vi "Process Command.vi"(8 "error in":errorcluster, 10 "message in":T1, 11 "lia rt in":refnum<class "Lock-In Amplifier Example RT.lvclass">) -> (0 "error out":errorcluster, 1 "send response":bool, 2 "message out":T1, 3 "lia rt out":refnum<class "Lock-In Amplifier Example RT.lvclass">)   [LabVIEW 2017, in "Lock-In Amplifier Example RT.lvclass"]
uses:
  Lock-In Amplifier Example RT.lvclass
  shared/Public/message.ctl
  host/Public/lock-in settings.ctl
  host/Public/pll settings.ctl
  Properties/FpgaSession_GET.vi
  interface/Interface FPGA/Properties/FpgaSession_GET.vi
  interface/Interface FPGA/LIA Host Interface FPGA.lvclass
  host/Lock-In Amplifier Example Host.lvlib
  shared/Lock-In Amplifier Example Shared.lvlib
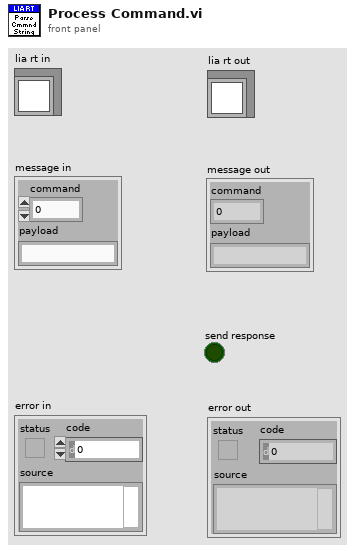
[diagram p1: front panel]
types:
  T1 = typedef "Lock-In Amplifier Example Shared.lvlib/message.ctl" = cluster{"command":u32, "payload":string}
  T2 = typedef "Lock-In Amplifier Example Host.lvlib/lock-in settings.ctl" = cluster{"decimation":i32, "source":i32, "carrier source":i32, "carrier":dbl}
  T3 = cluster{"instance":i32, "config":cluster{"config":T2, "record length":u32}}
  T4 = typedef "Lock-In Amplifier Example Host.lvlib/pll settings.ctl" = cluster{"source":i32, "q frequency":dbl}
  T5 = cluster{"instance":i32, "config":cluster{"carrier":dbl, "level":dbl}}
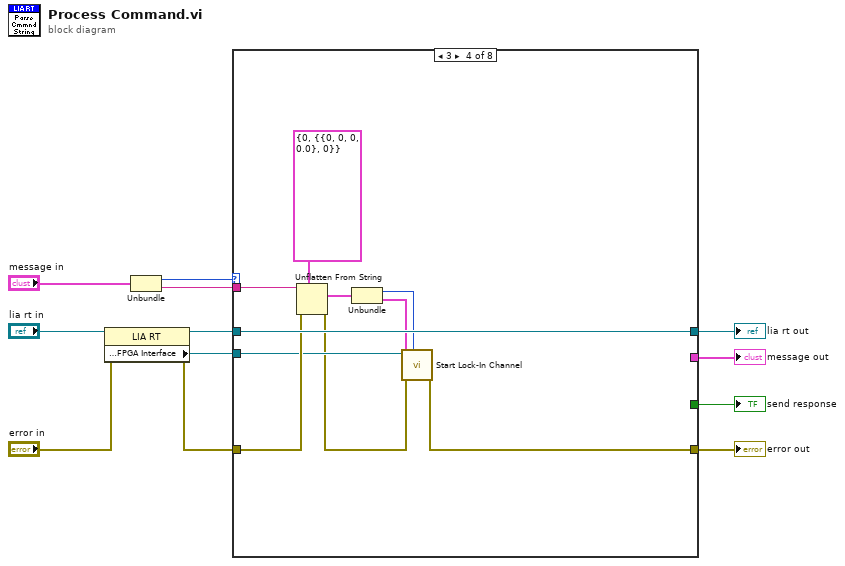
[diagram p0: block diagram]
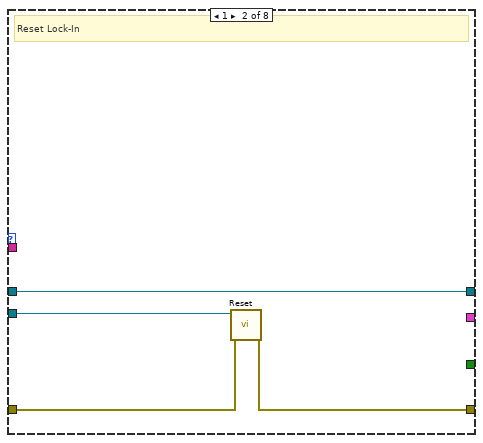
[diagram p3: hidden frame]
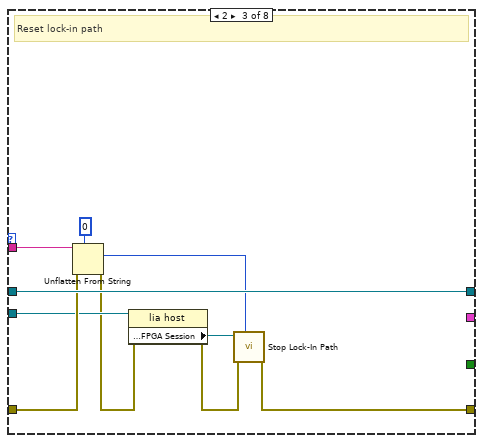
[diagram p4: hidden frame]
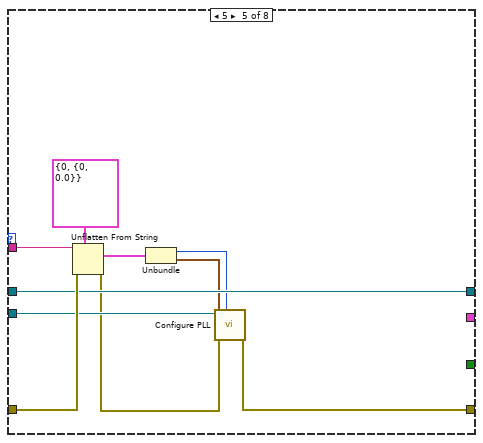
[diagram p5: hidden frame]
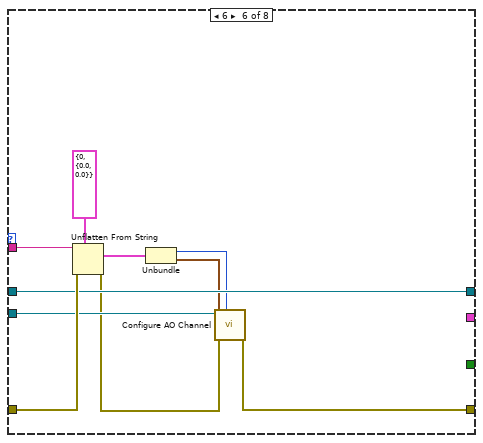
[diagram p6: hidden frame]
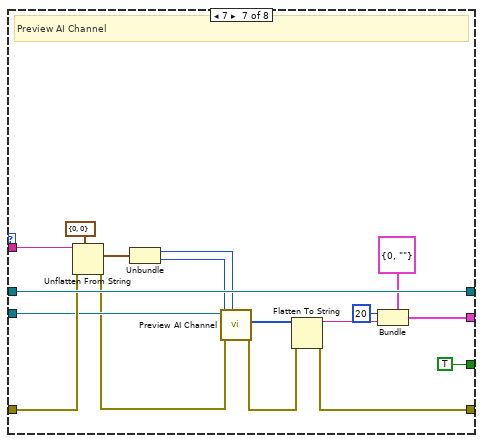
[diagram p7: hidden frame]
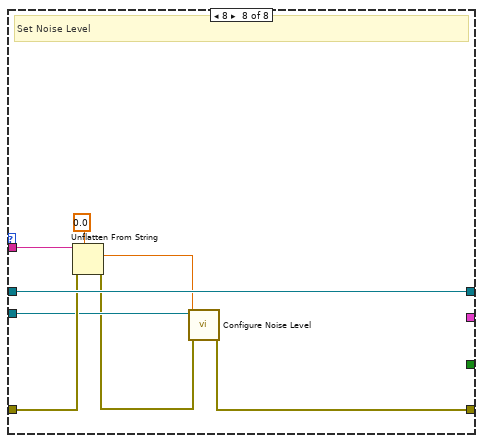
[diagram p8: hidden frame]
diagram:
  n1 = property class="LIA RT"(reference="lia rt in", error in="error in") -> (reference out=w8:refnum<class "Lock-In Amplifier Example RT.lvclass">, error out=w6:errorcluster, "Properties:FPGA Interface"=w5:refnum<class "LIA Host Interface FPGA.lvclass">)
  n2 = Unbundle("message in") -> ("command"=w11:u32, "payload"=w10:string)
  n3 = case shown="3" w11 {
    tunnel: w10 -> [_ _ w26 w37 w48 w58 w74 w82]
    tunnel: w8 -> [w14 w18 w28 w38 w43 w54 w75 w83]
    tunnel: w6 -> [w13 w16 w25 w36 w47 w57 w73 w81]
    tunnel: w5 -> [_ w17 w22 w35 w44 w55 w66 w80]
    tunnel: [w14 w18 w28 w38 w43 w54 w75 w83] -> w4
    tunnel: [w13 w15 w27 w33 w39 w51 w60 w76] -> w3
    tunnel: [_ _ _ _ _ _ w69 _] -> w2
    tunnel: [_ _ _ _ _ _ TRUE _] -> w1
    frame 0, Default {
    }
    frame 1 {
      # "Reset Lock-In"
      n4 = call-dynamic "Reset.vi"("error in"=w16, "host in"=w17) -> ("error out"=w15:errorcluster)  [unwired: 8 in, 1 out]
    }
    frame 2 {
      # "Reset lock-in path"
      n5 = Unflatten From String(type=0, binary string=w26, error in (no error)=w25) -> (value=w23:i32, error out=w21:errorcluster)  [unwired: 2 in, 1 out]
      n6 = property class="lia host"(reference=w22, error in=w21) -> (error out=w20:errorcluster, "Properties:FPGA Session"=w19:refnum<k20>)  [unwired: 1 out]
      n7 = call "Stop Lock-In Path.vi"("instance"=w23, "error in"=w20, "fpga session in"=w19) -> ("error out"=w27:errorcluster)  [unwired: 7 in, 1 out]
    }
    frame 3 {
      n8 = Unflatten From String(type=T3 {"instance"=0, "config"={"config"={"decimation"=0, "source"=0, "carrier source"=0, "carrier"=0.0}, "record length"=0}} ("output cluster"), binary string=w37, error in (no error)=w36) -> (value=w32:T3, error out=w34:errorcluster)  [unwired: 2 in, 1 out]
      n9 = Unbundle(w32) -> ("instance"=w31:i32, "config"=w30:cluster{"config":T2, "record length":u32})
      n10 = call-dynamic "Start Lock-In Channel.vi"("index"=w31, "error in"=w34, "config"=w30, "host in"=w35) -> ("error out"=w33:errorcluster)  [unwired: 6 in, 1 out]
    }
    frame 5 {
      n11 = Unflatten From String(type=cluster{"instance":i32, "config":T4} {"instance"=0, "config"={"source"=0, "q frequency"=0.0}}, binary string=w48, error in (no error)=w47) -> (value=w45:cluster{"instance":i32, "config":T4}, error out=w40:errorcluster)  [unwired: 2 in, 1 out]
      n12 = Unbundle(w45) -> ("instance"=w42:i32, "config"=w41:T4)
      n13 = call-dynamic "Configure PLL.vi"("index"=w42, "error in"=w40, "config"=w41, "host in"=w44) -> ("error out"=w39:errorcluster)  [unwired: 6 in, 1 out]
    }
    frame 6 {
      n14 = Unflatten From String(type=T5 {"instance"=0, "config"={"carrier"=0.0, "level"=0.0}} ("output cluster"), binary string=w58, error in (no error)=w57) -> (value=w56:T5, error out=w52:errorcluster)  [unwired: 2 in, 1 out]
      n15 = Unbundle(w56) -> ("instance"=w53:i32, "config"=w49:cluster{"carrier":dbl, "level":dbl})
      n16 = call-dynamic "Configure AO Channel.vi"("index"=w53, "error in"=w52, "config"=w49, "host in"=w55) -> ("error out"=w51:errorcluster)  [unwired: 6 in, 1 out]
    }
    frame 7 {
      # "Preview AI Channel"
      n17 = Unflatten From String(type=cluster{"instance":i32, "samples":u32} {"instance"=0, "samples"=0}, binary string=w74, error in (no error)=w73) -> (value=w71:cluster{"instance":i32, "samples":u32}, error out=w65:errorcluster)  [unwired: 2 in, 1 out]
      n18 = Unbundle(w71) -> ("instance"=w64:i32, "samples"=w63:u32)
      n19 = call-dynamic "Preview AI Channel.vi"("index"=w64, "error in"=w65, "samples"=w63, "host in"=w66) -> ("error out"=w61:errorcluster, "samples out"=w62:i16[])  [unwired: 5 in, 1 out]
      n20 = Flatten To String(anything=w62, error in (no error)=w61) -> (data string=w59:string, error out=w60:errorcluster)  [unwired: 2 in, 1 out]
      n21 = Bundle(cluster=T1 {"command"=0, "payload"=""} ("message"), "command"=u32 20, "payload"=w59) -> (w69:T1)
    }
    frame 8 {
      # "Set Noise Level"
      n22 = Unflatten From String(type=0.0, binary string=w82, error in (no error)=w81) -> (value=w77:dbl, error out=w79:errorcluster)  [unwired: 2 in, 1 out]
      n23 = call-dynamic "Configure Noise Level.vi"("error in"=w79, "level"=w77, "lia host in"=w80) -> ("error out"=w76:errorcluster)  [unwired: 7 in, 1 out]
    }
  }
  "error out" <- w3
  "lia rt out" <- w4
  "message out" <- w2
  "send response" <- w1
